vi "Video Processor Create.vi"(4 "Num Threads (-1: CPU count)":i32=-1, 5 "Identifier":string, 6 "Depth History Size (10)":i32=10, 7 "Open? (T)":bool=TRUE, 8 "error in (no error)":errorcluster, 9 "Sensor Index (0)":i32, 10 "Device Index (0)":i32, 11 "Video Processor in":refnum<class "Video Cam Processor.lvclass">) -> (0 "error out":errorcluster, 3 "Video Processor out":refnum<class "Video Cam Processor.lvclass">)   [LabVIEW 2018, in "Video Cam Processor.lvclass"]
uses:
  Video Cam Processor.lvclass
  C:/Users/aaron.jencks/Documents/GitHub/emerson_seed_object_detection/LabVIEW/Projects/Paul's Video Viewer/Classes/Realsense Cam Video File Wrapper/Realsense Cam File Wrapper.lvclass
  C:/Users/aaron.jencks/Documents/GitHub/emerson_seed_object_detection/LabVIEW/Projects/Paul's Video Viewer/Classes/Video File/Video File.lvclass
  Video Cam Processor.lvclass/Video Cam Processor.ctl
  <vilib>/vision/NI_Vision_Development_Module.lvlib
  Standard Averager/Standard Averager.lvclass
  Realsense Cam Video File Wrapper/Realsense Cam File Wrapper.lvclass
  Video File/Video File.lvclass
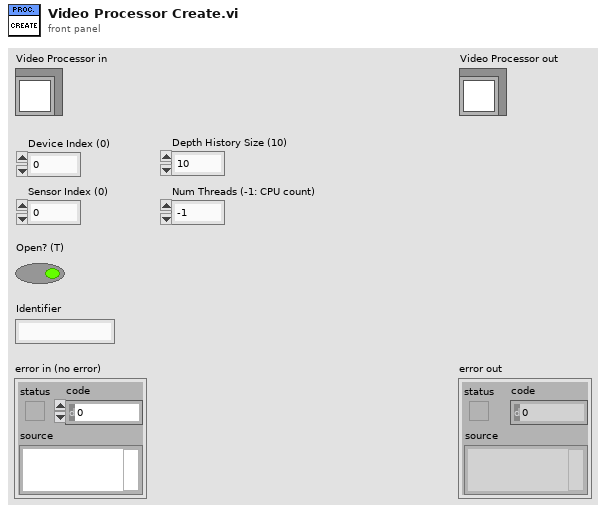
[diagram p1: front panel]
types:
  T1 = typedef "Image Type" = u32
  T2 = typedef "IMAQ Image.ctl" = refnum<image>
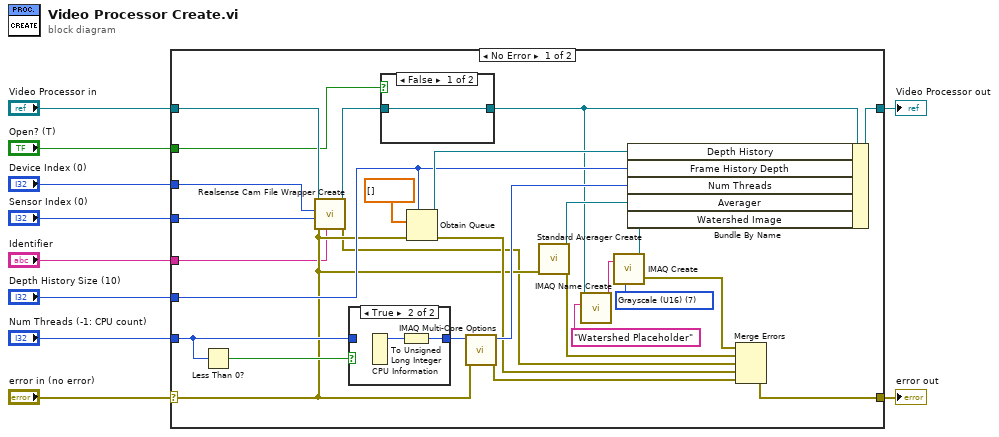
[diagram p0: block diagram]
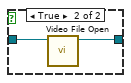
[diagram p2: hidden frame]
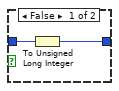
[diagram p3: hidden frame]
diagram:
  n1 = case shown="No Error" "error in (no error)" {
    selector: "error in (no error)" -> [w23 w46]
    tunnel: [w25 w46] -> w9
    tunnel: [w37 w45] -> w7
    tunnel: "Video Processor in" -> [w24 w45]
    tunnel: "Identifier" -> [w21 _]
    tunnel: "Depth History Size (10)" -> [w35 _]
    tunnel: "Num Threads (-1: CPU count)" -> [w31 _]
    tunnel: "Open? (T)" -> [w17 _]
    tunnel: "Device Index (0)" -> [w20 _]
    tunnel: "Sensor Index (0)" -> [w19 _]
    frame No Error {
      w11 = T1 7 items=["Grayscale (U8)", "Grayscale (I16)", "Grayscale (SGL)", "Complex (CSG)", "RGB (U32)", "HSL (U32)", "RGB (U64)", "Grayscale (U16)"] ("Image Type")
      n2 = Less Than 0?(x=w31) -> (x < 0?=w32:bool)
      n3 = call "Realsense Cam File Wrapper Create.vi"("Identifier"=w21, "error in (no error)"=w23, "Sensor Index (0)"=w19, "Device Index (0)"=w20, "Realsense Cam File Wrapper in"=w24) -> ("error out"=w22:errorcluster, "Realsense Cam File Wrapper out"=w18:refnum<class "Video Cam Processor.lvclass">)  [unwired: 5 in]
      n4 = case shown="True" w32 {
        tunnel: w31 -> [w42 _]
        tunnel: [w41 w43] -> w30
        frame False {
          n5 = To Unsigned Long Integer(number=w42) -> (unsigned 32bit integer=w41:u32)
        }
        frame True {
          n6 = CPU Information() -> (4:w44:i32)  [unwired: 3 out]
          n7 = To Unsigned Long Integer(number=w44) -> (unsigned 32bit integer=w43:u32)
        }
      }
      n8 = case shown="False" w17 {
        tunnel: w18 -> [w38 w40]
        tunnel: [w38 w39] -> w15
        frame False {
        }
        frame True {
          n9 = call-dynamic "Video File Open.vi"("Realsense Cam File Wrapper in"=w40) -> ("Realsense Cam File Wrapper out"=w39:refnum<class "Video Cam Processor.lvclass">)  [unwired: 9 in, 1 out]
        }
      }
      n10 = Obtain Queue(max queue size (-1, unlimited)=w35, element data type=dbl[] [], error in (no error)=w23) -> (queue out=w36:refnum<queue>, error out=w27:errorcluster)  [unwired: 2 in, 1 out]
      n11 = call "IMAQ Multi-Core Options"("error in (no error)"=w23, "Specified Number of Cores"=w30) -> ("error out"=w28:errorcluster, "Cores Utilized"=w33:u32)  [unwired: 8 in]
      n12 = call "Standard Averager Create.vi"("error in (no error)"=w23) -> ("error out"=w26:errorcluster, "Standard Averager out"=w29:refnum<class "Standard Averager.lvclass">)  [unwired: 9 in]
      n13 = call "IMAQ Name Create.vi"("Name (\"\")"="Watershed Placeholder" ("Name (\"\")"), "Video File in"=w15) -> ("Name Out"=w14:string)  [unwired: 7 in, 2 out]
      n14 = call "IMAQ Create"("Image Name"=w14, "Image Type"=w11) -> ("New Image"=w16:T2, "error out"=w12:errorcluster)  [unwired: 3 in]
      n15 = Bundle By Name(cluster=w15, "Depth History"=w36, "Frame History Depth"=w35, "Num Threads"=w33, "Averager"=w29, "Watershed Image"=w16) -> (w37:refnum<class "Video Cam Processor.lvclass">)
      n16 = Merge Errors(w12, w26, w22, w27, w28) -> (w25:errorcluster)
    }
    frame Error {
    }
  }
  "error out" <- w9
  "Video Processor out" <- w7
